vi "Send Fire Value to Cooker.vi"(8 "error in (no error)":errorcluster, 10 "Fire (%)":dbl min=0.0 max=100.0 format="%.2f", 11 "Oven Actor in":refnum<class "Oven Actor.lvclass">) -> (0 "error out":errorcluster, 3 "Oven Actor out":refnum<class "Oven Actor.lvclass">)   [LabVIEW 2021, in "Oven Actor.lvlib" / "Oven Actor.lvclass"]
uses:
  Oven Actor.lvclass
  <vilib>/ActorFramework/Actor/Actor.lvclass
  Cooker Actor/Cooker Actor Messages/Update Cooker Fire Msg/Update Cooker Fire Msg.lvclass
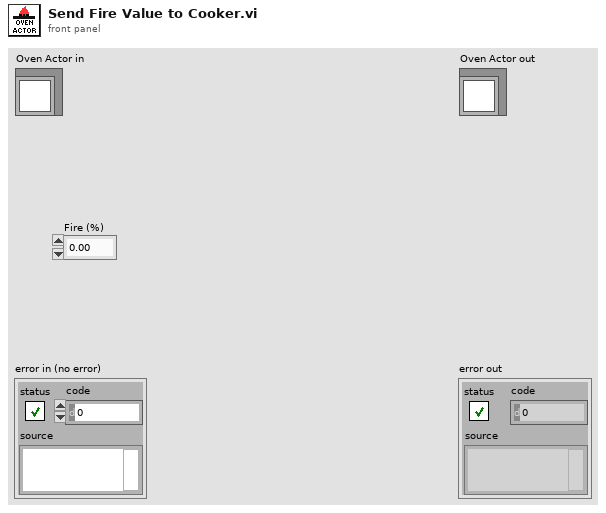
[diagram p1: front panel]
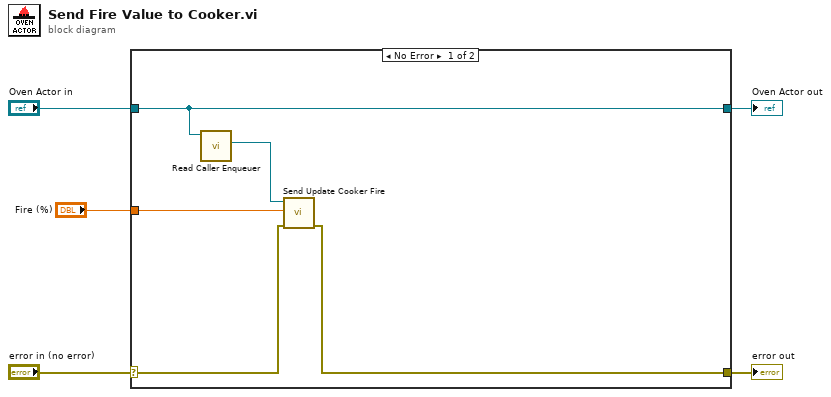
[diagram p0: block diagram]
diagram:
  n1 = case shown="No Error" "error in (no error)" {
    selector: "error in (no error)" -> [w7 w12]
    tunnel: [w6 w12] -> w4
    tunnel: [w9 w11] -> w2
    tunnel: "Oven Actor in" -> [w9 w11]
    tunnel: "Fire (%)" -> [w8 _]
    frame No Error {
      n2 = call <vilib>:"Read Caller Enqueuer.vi"("Actor"=w9) -> ("Caller Enqueuer"=w10:refnum<class "Message Enqueuer.lvclass">)  [unwired: 10 in]
      n3 = call "Send Update Cooker Fire.vi"("error in (no error)"=w7, "Fire (%)"=w8, "Message Enqueuer"=w10) -> ("error out"=w6:errorcluster)  [unwired: 7 in, 1 out]
    }
    frame Error {
    }
  }
  "error out" <- w4
  "Oven Actor out" <- w2
